vi "ElectrodeOn.vi"(8 "error in (no error)":errorcluster, 10 "Electrode On":bool=TRUE, 11 "Electrode in":refnum<class "Electrode.lvclass">) -> (0 "error out":errorcluster, 3 "Electrode out":refnum<class "Electrode.lvclass">)   [LabVIEW 2012, in "Electrode.lvclass"]
uses:
  Electrode.lvclass
  Electrode.lvclass/Electrode.ctl
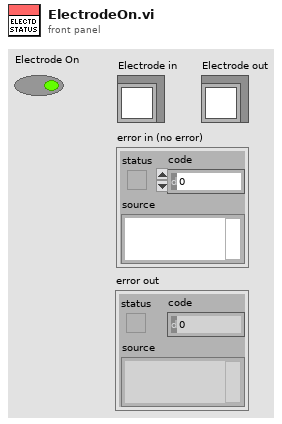
[diagram p1: front panel]
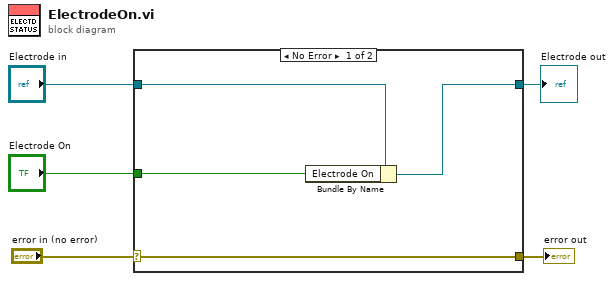
[diagram p0: block diagram]
diagram:
  n1 = case shown="No Error" "error in (no error)" {
    selector: "error in (no error)" -> [w9 w10]
    tunnel: [w9 w10] -> w4
    tunnel: [w7 w11] -> w2
    tunnel: "Electrode in" -> [w8 w11]
    tunnel: "Electrode On" -> [w6 _]
    frame No Error {
      n2 = Bundle By Name(cluster=w8, "Electrode On"=w6) -> (w7:refnum<class "Electrode.lvclass">)
    }
    frame Error {
    }
  }
  "error out" <- w4
  "Electrode out" <- w2
